vi "drawRoundRectangle.vi"(0 "reference":refnum<class "Graphics.lvclass">, 1 "rectangle":T1 {"height" format="%.2f"; "width" format="%.2f"; "y" format="%.2f"; "x" format="%.2f"}, 2 "lineWidth(1)":dbl=1.0 format="%.2f", 3 "color(if not used=default color)":u32=33554432 format="%.0x", 4 "fill?(F)":bool, 5 "error in (no error)":errorcluster, 7 "RoundRadius":i16=20, 9 "FillClor(if not used=BorderColorIsUsed,AutoFill)":u32=16777216 format="%.0x") -> (14 "reference out":refnum<class "Graphics.lvclass">, 19 "error out":errorcluster)   [LabVIEW 2016, in "Graphics.lvclass"]
uses:
  <resource>/Framework/Providers/Open_GDS/UML/Graphics_class/Graphics.lvclass
  <resource>/Framework/Providers/Open_GDS/UML/General/Rectangle/Rectangle Rectangle2D.ctl
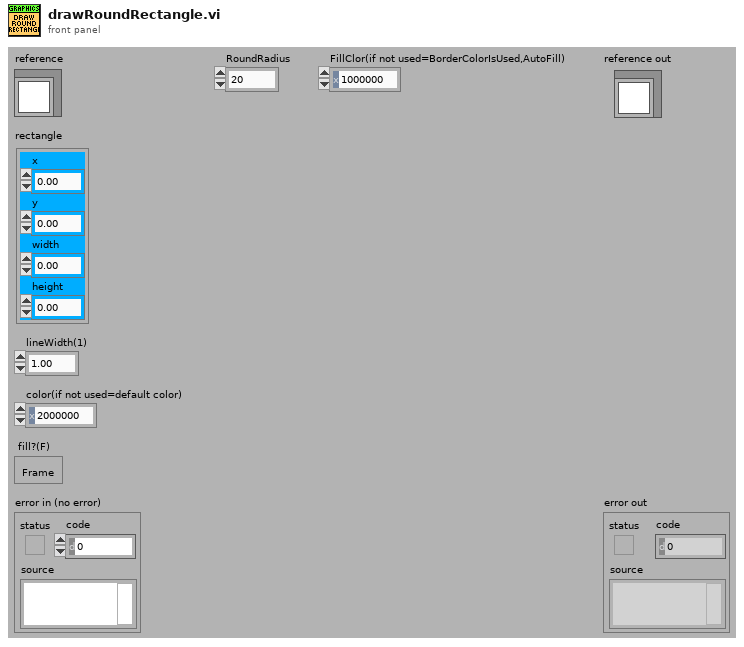
[diagram p1: front panel]
types:
  T1 = typedef "Rectangle Rectangle2D.ctl" = cluster{"x":dbl, "y":dbl, "width":dbl, "height":dbl}
  T2 = cluster{"Width":i16, "Style":enum32{"Solid", "Dash", "Dot", "DashDot", "DashDotDot"}}
  T3 = typedef "Graphics.lvclass/ObjectAttributes.ctl" = cluster{"drawColor":u32, "backgroundColor":u32, "font":T4, "fontType":T5, "picture":picture, "stroke":T6, "scaleX":dbl, "scaleY":dbl, "screenRef":refnum<vi>, "offsetX":dbl, "offsetY":dbl}
  T4 = typedef "Graphics.lvclass/FontType.ctl" = cluster{"Font Name:":string, "Size":i16, "Strikeout?":bool, "Italic?":bool, "Underline?":bool, "Outline?":bool, "Shadow?":bool, "Bold?":bool}
  T5 = typedef "Graphics.lvclass/LvFontType.ctl" = enum16{"User-specified Font", "Application Font", "System Font", "Dialog Font"}
  T6 = typedef "Graphics.lvclass/StrokeType.ctl" = enum16{"USE_DEFAULT", "SOLID", "DOTTED"}
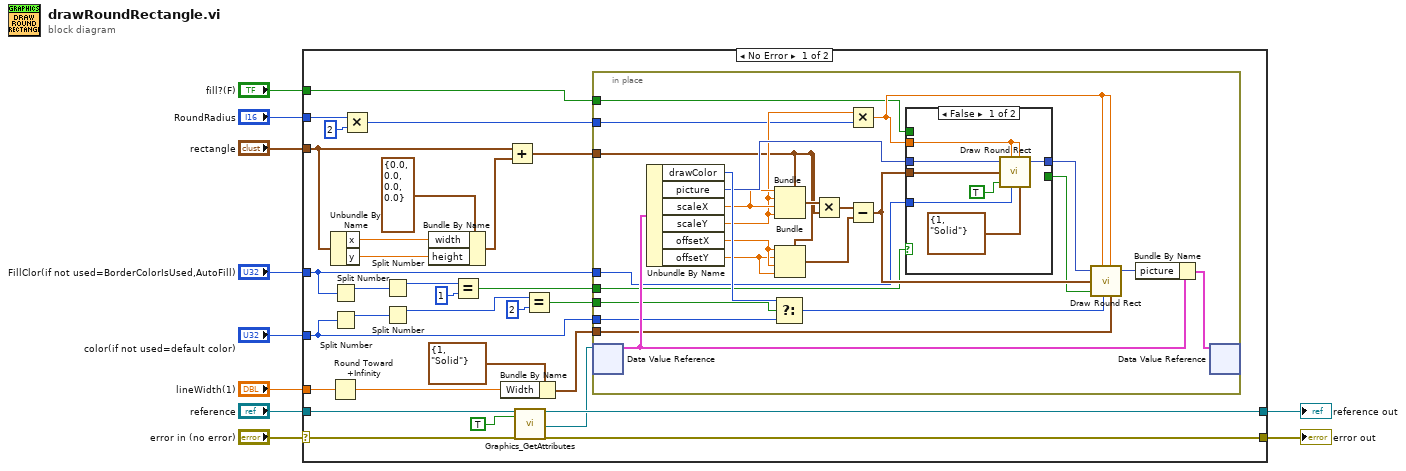
[diagram p0: block diagram]
diagram:
  n1 = case shown="No Error" "error in (no error)" {
    selector: "error in (no error)" -> [w37 w75]
    tunnel: "reference" -> [w40 w76]
    tunnel: [w39 w75] -> w9
    tunnel: [w38 w76] -> w8
    tunnel: "rectangle" -> [w36 _]
    tunnel: "lineWidth(1)" -> [w35 _]
    tunnel: "color(if not used=default color)" -> [w17 _]
    tunnel: "fill?(F)" -> [w14 _]
    tunnel: "RoundRadius" -> [w34 _]
    tunnel: "FillClor(if not used=BorderColorIsUsed,AutoFill)" -> [w13 _]
    frame No Error {
      n2 = Round Toward +Infinity(x=w35) -> (ceil(x): smallest int >= x=w21:dbl)
      n3 = Unbundle By Name(w36) -> ("x"=w29:dbl, "y"=w28:dbl)
      n4 = Split Number(x=w13) -> (hi(x)=w23:u16)  [unwired: 1 out]
      n5 = Split Number(x=w17) -> (hi(x)=w33:u16)  [unwired: 1 out]
      n6 = Multiply(x=w34, y=i16 2) -> (x*y=w12:i16)
      n7 = Split Number(x=w23) -> (hi(x)=w24:u8)  [unwired: 1 out]
      n8 = Split Number(x=w33) -> (hi(x)=w32:u8)  [unwired: 1 out]
      n9 = Bundle By Name(cluster=T1 {"x"=0.0, "y"=0.0, "width"=0.0, "height"=0.0} ("x"), "width"=w29, "height"=w28) -> (w27:T1)
      n10 = Equal?(x=w24, y=u8 1) -> (x = y?=w15:bool)
      n11 = Bundle By Name(cluster=T2 {"Width"=1, "Style"=enum."Solid"} ("pen"), "Width"=w21) -> (w18:T2)
      n12 = Add(x=w36, y=w27) -> (x+y=w11:T1)
      n13 = call <resource>:"Graphics_GetAttributes.vi"("reference in"=w40, "OnlyGetDvrReference(False)"=TRUE, "error in (no error)"=w37) -> ("reference out"=w38:refnum<class "Graphics.lvclass">, "DataRef"=w19:refnum<data-value>, "error out"=w39:errorcluster)  [unwired: 13 in, 1 out]
      n14 = Equal?(x=w32, y=u8 2) -> (x = y?=w16:bool)
      n15 = in-place {
        in-place-border: w18 -> [w51]
        in-place-border: w17 -> [w50]
        in-place-border: w16 -> [w49]
        in-place-border: w15 -> [w48]
        in-place-border: w14 -> [w47]
        in-place-border: w13 -> [w46]
        in-place-border: w12 -> [w44]
        in-place-border: w11 -> [w41]
        n16 = in-place-dvr #1(w19) -> (w65:T3)  [unwired: 1 out]
        n17 = Unbundle By Name(w65) -> ("drawColor"=w62:u32, "picture"=w61:picture, "scaleX"=w60:dbl, "scaleY"=w59:dbl, "offsetX"=w58:dbl, "offsetY"=w57:dbl)
        n18 = Select(t=w62, s=w49, f=w50) -> (s? t:f=w52:u32)
        n19 = Bundle(cluster=w41, "x"=w60, "y"=w59, "width"=w60, "height"=w59) -> (w45:T1)
        n20 = Bundle(cluster=w41, "x"=w58, "y"=w57, "width"=w58, "height"=w57) -> (w43:T1)
        n21 = Multiply(x=w45, y=w41) -> (x*y=w42:T1)
        n22 = Multiply(x=w59, y=w44) -> (x*y=w55:dbl)
        n23 = Subtract(x=w42, y=w43) -> (x-y=w54:T1)
        n24 = case shown="False" w48 {
          tunnel: w47 -> [_ w74]
          tunnel: [_ w74] -> w53
          tunnel: w61 -> [w72 w73]
          tunnel: [w71 w73] -> w56
          tunnel: w46 -> [w69 _]
          tunnel: w55 -> [w70 _]
          tunnel: w54 -> [w67 _]
          frame False {
            n25 = call <vilib>:"Draw Round Rect.vi"("picture"=w72, "oval width"=w70, "rect"=w67, "fill?(F)"=TRUE, "color(black)"=w69, "oval height"=w70, "pen"=T2 {"Width"=1, "Style"=enum."Solid"}) -> ("new picture"=w71:picture)  [unwired: 2 out]
          }
          frame True {
          }
        }
        n26 = call <vilib>:"Draw Round Rect.vi"("picture"=w56, "oval width"=w55, "rect"=w54, "fill?(F)"=w53, "color(black)"=w52, "oval height"=w55, "pen"=w51) -> ("new picture"=w64:picture)  [unwired: 2 out]
        n27 = Bundle By Name(cluster=w65, "picture"=w64) -> (w63:T3)
        n28 = in-place-dvr #1(w63) -> ()  [unwired: 2 out]
      }
    }
    frame Error {
    }
  }
  "reference out" <- w8
  "error out" <- w9
